vi "CheckBoundsAndIncrement.vi"(4 "error in":errorcluster, 6 "Rectangle In":T1, 7 "Increment":T1) -> (0 "error out":errorcluster, 3 "Rectangle Out":T1)   [LabVIEW 2021, in "Ants.lvclass"]
doc: "This VI adds <b>Increment</b> to <b>Rectangle In</b>, checks that both axes have at least 1 corner in the range 1-31 (i.e. rectangle in valid range), and returns the resulting rectangle.\n\nIf the resulting rectangle is invalid, this VI returns <b>Rectangle Input</b> unmodified."
uses:
  <resource>/plugins/NIIconEditor/Class/Ants/Ants.lvclass
  <resource>/plugins/NIIconEditor/Class/Ants/Ants.lvclass/Ants.ctl
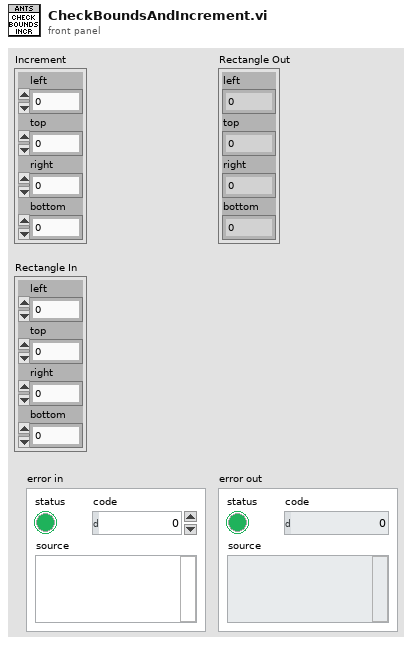
[diagram p1: front panel]
types:
  T1 = cluster{"left":i16, "top":i16, "right":i16, "bottom":i16}
  T2 = cluster{"left":bool, "top":bool, "right":bool, "bottom":bool}
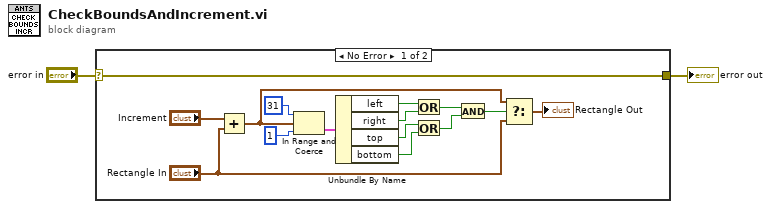
[diagram p0: block diagram]
diagram:
  n1 = case shown="No Error" "error in" {
    selector: "error in" -> [w6 w18]
    tunnel: [w6 w18] -> w1
    frame No Error {
      n2 = Add(x="Increment", y="Rectangle In") -> (x+y=w3:T1)
      n3 = In Range and Coerce(upper limit=31, x=w3, lower limit=1) -> (In Range?=w15:T2)  [unwired: 1 out]
      n4 = Unbundle By Name(w15) -> ("left"=w14:bool, "right"=w13:bool, "top"=w12:bool, "bottom"=w11:bool)
      n5 = Or(x=w14, y=w13) -> (x .or. y?=w10:bool)
      n6 = Or(x=w12, y=w11) -> (x .or. y?=w9:bool)
      n7 = And(x=w10, y=w9) -> (x .and. y?=w8:bool)
      n8 = Select(t=w3, s=w8, f="Rectangle In") -> (s? t:f=→"Rectangle Out":T1)
    }
    frame Error {
    }
  }
  "error out" <- w1
